vi "MakeDataFile.vi"(11 "created path":path) -> (3 "Path":path)   [LabVIEW 2018]
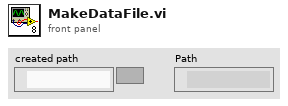
[diagram p1: front panel]
types:
  T1 = enum16{"open", "replace", "create", "open or create", "replace or create", "replace or create with confirmation"}
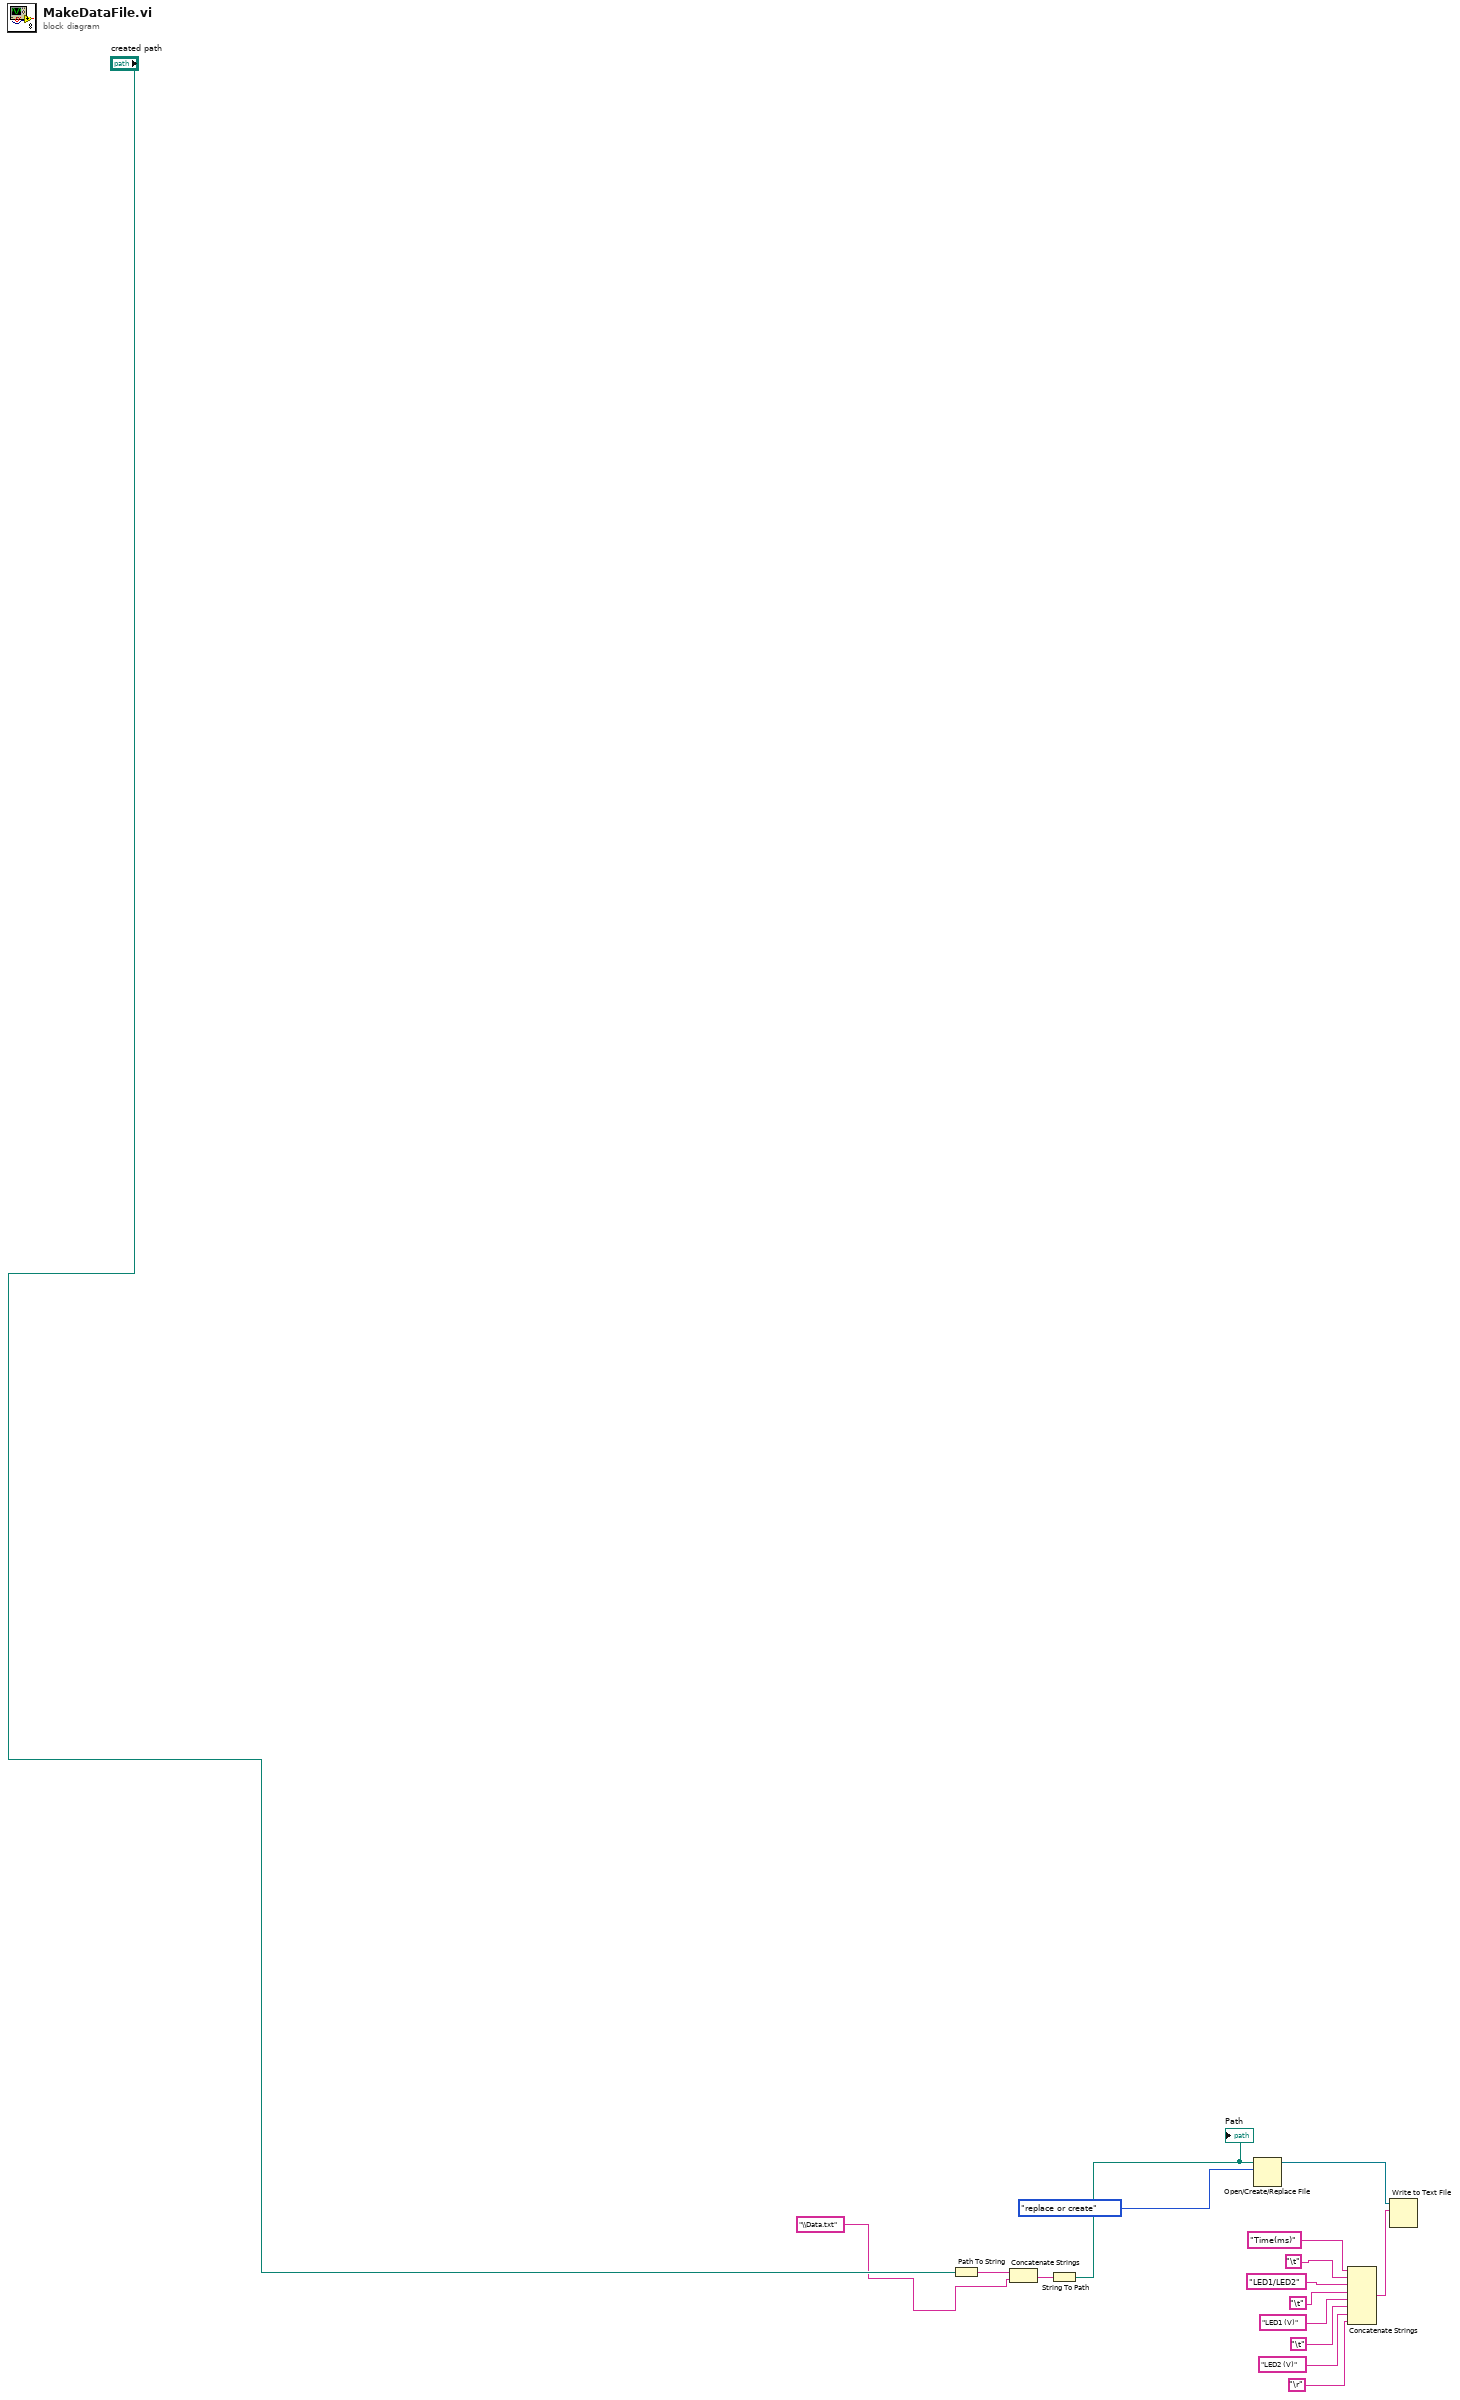
[diagram p0: block diagram]
diagram:
  n1 = Path To String(path="created path") -> (string=w12:string)
  n2 = Concatenate Strings(w12, "\\Data.txt") -> (w13:string)
  n3 = String To Path(string=w13) -> (path=w15:path)
  "Path" <- w15
  n4 = Open/Create/Replace File(file path (use dialog)=w15, operation (0:open)=T1."replace or create") -> (refnum out=w10:refnum<file>)  [unwired: 4 in, 2 out]
  n5 = Concatenate Strings("Time(ms)" ("text"), "\t", "LED1/LED2" ("text"), "\t", "LED1 (V)" ("text"), "\t", "LED2 (V)" ("text"), "\r") -> (w8:string)
  n6 = Write to Text File(file (use dialog)=w10, text=w8) -> ()  [unwired: 2 in, 3 out]
